vi "modbus slave全局.vi"() -> ()   [LabVIEW 2016, in "MB SLAVE.lvlib"]
uses:
  MB SLAVE.lvlib
  <vilib>/Plasmionique/MB Master/MB_Master/MB_Master.lvclass
panel:
  in  "选项卡控件":T1(tab)
  in  "与CODMn交互全局":T2 {"加标回收启动时间" format="%<%Y/%m/%d %H:%M:%S>T"; "水样启动时间" format="%<%Y/%m/%d %H:%M:%S>T"}
  in  "与氨氮交互全局":T3 {"状态告警区"."工作状态" items=["空闲"=0, "水样测试"=1, "标样核查"=2, "零点核查"=3, "跨度核查"=4, "空白测试"=5, "平行样测试"=6, "加标回收"=7, "空白校准"=8, "标样校准"=9, "初始化（清洗）"=10, "单步调试"=254, "简易流程"=255]; "状态告警区"."告警代码" items=["无告警", "缺试剂告警", "缺水样告警", "缺蒸馏水告警", "缺标液告警", "仪表漏液告警", "标定异常告警", "超量程告警", "加热异常", "低试剂预警", "超上限告警", "超下限告警", "仪表内部其他异常", "滴定异常告警", "电极异常告警", "量程切换告警", "参数设置告警", "PH电极电位异常", "电导率电极异常", "浊度光度异常", "溶解氧电极异常", "溶解氧光强异常", "温度异常告警", "PH异常告警", "溶解氧异常告警", "电导率异常告警", "浊度异常告警", "叶绿素异常告警", "藻密度异常告警", "蓝绿藻异常告警", "ORP异常告警", "氨氮异常告警", "清洁刷异常告警", "SD卡异常告警", "蓝牙异常告警", "Wifi异常告警", "流程异常告警"]; "状态告警区"."故障代码" items=["无故障", "电机故障", "温度故障", "通讯故障", "滴定故障"]}
  in  "与总磷交互全局":T4 {"状态告警区"."工作状态" items=["空闲"=0, "水样测试"=1, "标样核查"=2, "零点核查"=3, "跨度核查"=4, "空白测试"=5, "平行样测试"=6, "加标回收"=7, "空白校准"=8, "标样校准"=9, "初始化（清洗）"=10, "单步调试"=254, "简易流程"=255]; "状态告警区"."告警代码" items=["无告警", "缺试剂告警", "缺水样告警", "缺蒸馏水告警", "缺标液告警", "仪表漏液告警", "标定异常告警", "超量程告警", "加热异常", "低试剂预警", "超上限告警", "超下限告警", "仪表内部其他异常", "滴定异常告警", "电极异常告警", "量程切换告警", "参数设置告警", "PH电极电位异常", "电导率电极异常", "浊度光度异常", "溶解氧电极异常", "溶解氧光强异常", "温度异常告警", "PH异常告警", "溶解氧异常告警", "电导率异常告警", "浊度异常告警", "叶绿素异常告警", "藻密度异常告警", "蓝绿藻异常告警", "ORP异常告警", "氨氮异常告警", "清洁刷异常告警", "SD卡异常告警", "蓝牙异常告警", "Wifi异常告警", "流程异常告警"]; "状态告警区"."故障代码" items=["无故障", "电机故障", "温度故障", "通讯故障", "滴定故障"]}
  in  "与总氮交互全局":T5 {"状态告警区"."工作状态" items=["空闲"=0, "水样测试"=1, "标样核查"=2, "零点核查"=3, "跨度核查"=4, "空白测试"=5, "平行样测试"=6, "加标回收"=7, "空白校准"=8, "标样校准"=9, "初始化（清洗）"=10, "单步调试"=254, "简易流程"=255]; "状态告警区"."告警代码" items=["无告警", "缺试剂告警", "缺水样告警", "缺蒸馏水告警", "缺标液告警", "仪表漏液告警", "标定异常告警", "超量程告警", "加热异常", "低试剂预警", "超上限告警", "超下限告警", "仪表内部其他异常", "滴定异常告警", "电极异常告警", "量程切换告警", "参数设置告警", "PH电极电位异常", "电导率电极异常", "浊度光度异常", "溶解氧电极异常", "溶解氧光强异常", "温度异常告警", "PH异常告警", "溶解氧异常告警", "电导率异常告警", "浊度异常告警", "叶绿素异常告警", "藻密度异常告警", "蓝绿藻异常告警", "ORP异常告警", "氨氮异常告警", "清洁刷异常告警", "SD卡异常告警", "蓝牙异常告警", "Wifi异常告警", "流程异常告警"]; "状态告警区"."故障代码" items=["无故障", "电机故障", "温度故障", "通讯故障", "滴定故障"]}
  in  "与CODCr交互全局":T6 {"状态告警区"."工作状态" items=["空闲"=0, "水样测试"=1, "标样核查"=2, "零点核查"=3, "跨度核查"=4, "空白测试"=5, "平行样测试"=6, "加标回收"=7, "空白校准"=8, "标样校准"=9, "初始化（清洗）"=10, "单步调试"=254, "简易流程"=255]; "状态告警区"."告警代码" items=["无告警", "缺试剂告警", "缺水样告警", "缺蒸馏水告警", "缺标液告警", "仪表漏液告警", "标定异常告警", "超量程告警", "加热异常", "低试剂预警", "超上限告警", "超下限告警", "仪表内部其他异常", "滴定异常告警", "电极异常告警", "量程切换告警", "参数设置告警", "PH电极电位异常", "电导率电极异常", "浊度光度异常", "溶解氧电极异常", "溶解氧光强异常", "温度异常告警", "PH异常告警", "溶解氧异常告警", "电导率异常告警", "浊度异常告警", "叶绿素异常告警", "藻密度异常告警", "蓝绿藻异常告警", "ORP异常告警", "氨氮异常告警", "清洁刷异常告警", "SD卡异常告警", "蓝牙异常告警", "Wifi异常告警", "流程异常告警"]; "状态告警区"."故障代码" items=["无故障", "电机故障", "温度故障", "通讯故障", "滴定故障"]}
  in  "与多参数交互":T7={"pH"=TRUE, "DO"=TRUE, "Turb"=TRUE, "Cond"=TRUE, "Temp"=TRUE, "叶绿素a启用"=FALSE, "蓝绿藻"=FALSE, "藻密度"=FALSE, "orp"=FALSE}
  in  "与超标留样交互":T8
  in  "与系统交互":T9={"运行模式"=enum."维护模式", "运行间隔"=4, "流程运行中"=FALSE, "自动运行启动参数"={"氨氮"=FALSE, "总磷"=FALSE, "总氮"=FALSE, "多参数"=FALSE, "CODmn"=FALSE, "CODCr"=FALSE, "氟化物"=FALSE, "超标留样"=FALSE, "重金属"=FALSE, "挥发酚"=FALSE}, "SYSTEM Interface.总磷总氮类型"=enum."单模块", "多参数运行间隔"=4, "配水时间"=0.0, "沉淀时间"=0.0, "清洗时间"=0.0, "关键参数改变"=FALSE, "温度告警"=FALSE, "湿度告警"=FALSE, "烟感告警"=FALSE, "水浸告警"=FALSE, "开门告警"=FALSE, "SystemTask"=enum."停机", "PumpState"=enum."--", "除藻选择"=enum."不开除藻", "报警信息"=enum."无报警", "软件升级"=FALSE, "固件升级"=enum."无", "数据传输软件升级"=FALSE, "数采仪软件版本"=""} {"多参数运行间隔" min=1 max=24; "运行间隔" min=1 max=24}
  in  "Pump MB session in":refnum<class "MB_Master.lvclass">
  in  "NH3N session in":refnum<class "MB_Master.lvclass">
  in  "TP MB session in":refnum<class "MB_Master.lvclass">
  in  "TN MB session in":refnum<class "MB_Master.lvclass">
  in  "CODMn MB session in":refnum<class "MB_Master.lvclass">
  in  "CODCr MB session in":refnum<class "MB_Master.lvclass">
  in  "氟化物 MB session in":refnum<class "MB_Master.lvclass">
  in  "执行结果反馈":u16[](array[numeric])
  # "氨氮"
  # "总磷总氮"
  # "总氮"
  # "CODmn"
  # "CODCr"
  # "超标留样"
  # "多参数"
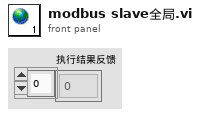
[diagram p1: front panel]
types:
  T1 = enum32{"CODMn", "氨氮", "总磷", "总氮", "CODCr", "多参数", "超标留样", "系统"}
  T2 = typedef "CODMn交互.ctl" = cluster{"COD浓度（mg/L)":dbl, "水样启动时间":timestamp, "加标回收启动时间":timestamp, "CODMn工作状态":enum16{"空闲", "水样测试", "标样核查", "零点核查", "跨度核查", "空白测试", "平行样测试", "加标回收", "空白校准", "标样校准", "初始化（清洗）"}, "多列列表框":i32, "平台试剂余量百分比":sgl, "关键参数":cluster{"测量量程":dbl, "测量精度":dbl, "测量间隔":dbl, "消解温度":dbl, "消解时长":dbl, "空白校准时间":timestamp, "曲线截距":dbl, "曲线斜率":dbl, "测量检出限":dbl, "测量信号值":dbl, "线性相关系数":dbl, "二次多项式系数":dbl, "标样校准时间":timestamp, "稀释倍数":dbl, "三项式系数":dbl, "空白标定系数":dbl, "量程系数":dbl, "F0/ORPA":dbl, "F1/ORPB":dbl, "F2/ORPK":dbl, "F3":dbl, "F4":dbl, "F5":dbl, "F6":dbl, "F7":dbl, "X0/滴定数":dbl, "量程":dbl}, "关键参数改变":bool, "校准信息":cluster{"低标液1浓度":dbl, "低标液1信号值":dbl, "低标液1启用":u16, "低标液2浓度":dbl, "低标液2信号值":dbl, "低标液2启用":u16, "低标液3浓度":dbl, "低标液3信号值":dbl, "低标液3启用":u16, "低标液4浓度":dbl, "低标液4信号值":dbl, "低标液4启用":u16, "低标液5浓度":dbl, "低标液5信号值":dbl, "低标液5启用":u16, "高标液1浓度":dbl, "高标液1信号值":dbl, "高标液1启用":u16, "高标液2浓度":dbl, "高标液2信号值":dbl, "高标液2启用":u16, "高标液3浓度":dbl, "高标液3信号值":dbl, "高标液3启用":u16, "高标液4浓度":dbl, "高标液4信号值":dbl, "高标液4启用":u16, "高标液5浓度":dbl, "高标液5信号值":dbl, "高标液5启用":u16, "低斜率":dbl, "低截距":dbl, "低二次多项式系数":dbl, "低线性相关系数":dbl, "高斜率":dbl, "高截距":dbl, "高二次多项式系数":dbl, "高线性相关系数":dbl}, "校准信息改变":bool, "固件版本号":string}
  T3 = typedef "氨氮交互.ctl" = cluster{"状态告警区":cluster{"系统时间":timestamp, "工作状态":u16, "测量模式":enum16{"待机", "连续模式", "周期模式", "定点模式", "受控模式", "手动模式"}, "告警代码":u16, "故障代码":u16, "日志代码":u16, "软件版本":u16, "F0":sgl, "F1":sgl, "F2":sgl, "F3":sgl, "T":sgl, "H":sgl, "id":u16, "flowid":u16, "量程":u16, "总磷控温温度1":sgl, "营养盐控温温度2":sgl, "ADC":sgl}, "平台试剂余量百分比":sgl, "关键参数":cluster{"测量量程":dbl, "测量精度":dbl, "测量间隔":dbl, "消解温度":dbl, "消解时长":dbl, "空白校准时间":timestamp, "曲线截距":dbl, "曲线斜率":dbl, "测量检出限":dbl, "测量信号值":dbl, "线性相关系数":dbl, "二次多项式系数":dbl, "标样校准时间":timestamp, "稀释倍数":dbl, "三项式系数":dbl, "空白标定系数":dbl, "量程系数":dbl, "F0/ORPA":dbl, "F1/ORPB":dbl, "F2/ORPK":dbl, "F3":dbl, "F4":dbl, "F5":dbl, "F6":dbl, "F7":dbl, "X0/滴定数":dbl, "量程":dbl}, "关键参数改变":bool, "校准信息":cluster{"低标液1浓度":dbl, "低标液1信号值":dbl, "低标液1启用":u16, "低标液2浓度":dbl, "低标液2信号值":dbl, "低标液2启用":u16, "低标液3浓度":dbl, "低标液3信号值":dbl, "低标液3启用":u16, "低标液4浓度":dbl, "低标液4信号值":dbl, "低标液4启用":u16, "低标液5浓度":dbl, "低标液5信号值":dbl, "低标液5启用":u16, "高标液1浓度":dbl, "高标液1信号值":dbl, "高标液1启用":u16, "高标液2浓度":dbl, "高标液2信号值":dbl, "高标液2启用":u16, "高标液3浓度":dbl, "高标液3信号值":dbl, "高标液3启用":u16, "高标液4浓度":dbl, "高标液4信号值":dbl, "高标液4启用":u16, "高标液5浓度":dbl, "高标液5信号值":dbl, "高标液5启用":u16, "低斜率":dbl, "低截距":dbl, "低二次多项式系数":dbl, "低线性相关系数":dbl, "高斜率":dbl, "高截距":dbl, "高二次多项式系数":dbl, "高线性相关系数":dbl}, "校准信息改变":bool, "固件版本号":string}
  T4 = typedef "总磷交互.ctl" = cluster{"状态告警区":cluster{"系统时间":timestamp, "工作状态":u16, "测量模式":enum16{"待机", "连续模式", "周期模式", "定点模式", "受控模式", "手动模式"}, "告警代码":u16, "故障代码":u16, "日志代码":u16, "软件版本":u16, "F0":sgl, "F1":sgl, "F2":sgl, "F3":sgl, "T":sgl, "H":sgl, "id":u16, "flowid":u16, "量程":u16, "总磷控温温度1":sgl, "营养盐控温温度2":sgl, "ADC":sgl}, "平台试剂余量百分比":sgl, "关键参数":cluster{"测量量程":dbl, "测量精度":dbl, "测量间隔":dbl, "消解温度":dbl, "消解时长":dbl, "空白校准时间":timestamp, "曲线截距":dbl, "曲线斜率":dbl, "测量检出限":dbl, "测量信号值":dbl, "线性相关系数":dbl, "二次多项式系数":dbl, "标样校准时间":timestamp, "稀释倍数":dbl, "三项式系数":dbl, "空白标定系数":dbl, "量程系数":dbl, "F0/ORPA":dbl, "F1/ORPB":dbl, "F2/ORPK":dbl, "F3":dbl, "F4":dbl, "F5":dbl, "F6":dbl, "F7":dbl, "X0/滴定数":dbl, "量程":dbl}, "关键参数改变":bool, "校准信息":cluster{"低标液1浓度":dbl, "低标液1信号值":dbl, "低标液1启用":u16, "低标液2浓度":dbl, "低标液2信号值":dbl, "低标液2启用":u16, "低标液3浓度":dbl, "低标液3信号值":dbl, "低标液3启用":u16, "低标液4浓度":dbl, "低标液4信号值":dbl, "低标液4启用":u16, "低标液5浓度":dbl, "低标液5信号值":dbl, "低标液5启用":u16, "高标液1浓度":dbl, "高标液1信号值":dbl, "高标液1启用":u16, "高标液2浓度":dbl, "高标液2信号值":dbl, "高标液2启用":u16, "高标液3浓度":dbl, "高标液3信号值":dbl, "高标液3启用":u16, "高标液4浓度":dbl, "高标液4信号值":dbl, "高标液4启用":u16, "高标液5浓度":dbl, "高标液5信号值":dbl, "高标液5启用":u16, "低斜率":dbl, "低截距":dbl, "低二次多项式系数":dbl, "低线性相关系数":dbl, "高斜率":dbl, "高截距":dbl, "高二次多项式系数":dbl, "高线性相关系数":dbl}, "校准信息改变":bool, "固件版本号":string}
  T5 = typedef "总氮交互.ctl" = cluster{"状态告警区":cluster{"系统时间":timestamp, "工作状态":u16, "测量模式":enum16{"待机", "连续模式", "周期模式", "定点模式", "受控模式", "手动模式"}, "告警代码":u16, "故障代码":u16, "日志代码":u16, "软件版本":u16, "F0":sgl, "F1":sgl, "F2":sgl, "F3":sgl, "T":sgl, "H":sgl, "id":u16, "flowid":u16, "量程":u16, "总磷控温温度1":sgl, "营养盐控温温度2":sgl, "ADC":sgl}, "平台试剂余量百分比":sgl, "关键参数":cluster{"测量量程":dbl, "测量精度":dbl, "测量间隔":dbl, "消解温度":dbl, "消解时长":dbl, "空白校准时间":timestamp, "曲线截距":dbl, "曲线斜率":dbl, "测量检出限":dbl, "测量信号值":dbl, "线性相关系数":dbl, "二次多项式系数":dbl, "标样校准时间":timestamp, "稀释倍数":dbl, "三项式系数":dbl, "空白标定系数":dbl, "量程系数":dbl, "F0/ORPA":dbl, "F1/ORPB":dbl, "F2/ORPK":dbl, "F3":dbl, "F4":dbl, "F5":dbl, "F6":dbl, "F7":dbl, "X0/滴定数":dbl, "量程":dbl}, "关键参数改变":bool, "校准信息":cluster{"低标液1浓度":dbl, "低标液1信号值":dbl, "低标液1启用":u16, "低标液2浓度":dbl, "低标液2信号值":dbl, "低标液2启用":u16, "低标液3浓度":dbl, "低标液3信号值":dbl, "低标液3启用":u16, "低标液4浓度":dbl, "低标液4信号值":dbl, "低标液4启用":u16, "低标液5浓度":dbl, "低标液5信号值":dbl, "低标液5启用":u16, "高标液1浓度":dbl, "高标液1信号值":dbl, "高标液1启用":u16, "高标液2浓度":dbl, "高标液2信号值":dbl, "高标液2启用":u16, "高标液3浓度":dbl, "高标液3信号值":dbl, "高标液3启用":u16, "高标液4浓度":dbl, "高标液4信号值":dbl, "高标液4启用":u16, "高标液5浓度":dbl, "高标液5信号值":dbl, "高标液5启用":u16, "低斜率":dbl, "低截距":dbl, "低二次多项式系数":dbl, "低线性相关系数":dbl, "高斜率":dbl, "高截距":dbl, "高二次多项式系数":dbl, "高线性相关系数":dbl}, "校准信息改变":bool, "固件版本号":string}
  T6 = typedef "CODCr交互.ctl" = cluster{"状态告警区":cluster{"系统时间":timestamp, "工作状态":u16, "测量模式":enum16{"待机", "连续模式", "周期模式", "定点模式", "受控模式", "手动模式"}, "告警代码":u16, "故障代码":u16, "日志代码":u16, "软件版本":u16, "F0":sgl, "F1":sgl, "F2":sgl, "F3":sgl, "T":sgl, "H":sgl, "id":u16, "flowid":u16, "量程":u16, "总磷控温温度1":sgl, "营养盐控温温度2":sgl, "ADC":sgl}, "平台试剂余量百分比":sgl, "关键参数":cluster{"测量量程":dbl, "测量精度":dbl, "测量间隔":dbl, "消解温度":dbl, "消解时长":dbl, "空白校准时间":timestamp, "曲线截距":dbl, "曲线斜率":dbl, "测量检出限":dbl, "测量信号值":dbl, "线性相关系数":dbl, "二次多项式系数":dbl, "标样校准时间":timestamp, "稀释倍数":dbl, "三项式系数":dbl, "空白标定系数":dbl, "量程系数":dbl, "F0/ORPA":dbl, "F1/ORPB":dbl, "F2/ORPK":dbl, "F3":dbl, "F4":dbl, "F5":dbl, "F6":dbl, "F7":dbl, "X0/滴定数":dbl, "量程":dbl}, "关键参数改变":bool, "校准信息":cluster{"低标液1浓度":dbl, "低标液1信号值":dbl, "低标液1启用":u16, "低标液2浓度":dbl, "低标液2信号值":dbl, "低标液2启用":u16, "低标液3浓度":dbl, "低标液3信号值":dbl, "低标液3启用":u16, "低标液4浓度":dbl, "低标液4信号值":dbl, "低标液4启用":u16, "低标液5浓度":dbl, "低标液5信号值":dbl, "低标液5启用":u16, "高标液1浓度":dbl, "高标液1信号值":dbl, "高标液1启用":u16, "高标液2浓度":dbl, "高标液2信号值":dbl, "高标液2启用":u16, "高标液3浓度":dbl, "高标液3信号值":dbl, "高标液3启用":u16, "高标液4浓度":dbl, "高标液4信号值":dbl, "高标液4启用":u16, "高标液5浓度":dbl, "高标液5信号值":dbl, "高标液5启用":u16, "低斜率":dbl, "低截距":dbl, "低二次多项式系数":dbl, "低线性相关系数":dbl, "高斜率":dbl, "高截距":dbl, "高二次多项式系数":dbl, "高线性相关系数":dbl}, "校准信息改变":bool, "固件版本号":string}
  T7 = typedef "多参数交互.ctl" = cluster{"pH":bool, "DO":bool, "Turb":bool, "Cond":bool, "Temp":bool, "叶绿素a启用":bool, "蓝绿藻":bool, "藻密度":bool, "orp":bool}
  T8 = typedef "超标留样交互.ctl" = cluster{"当前瓶号":u16}
  T9 = typedef "系统交互.ctl" = cluster{"运行模式":enum16{"维护模式", "常规模式", "应急模式", "质控模式", "性能测试"}, "运行间隔":i16, "流程运行中":bool, "自动运行启动参数":T10, "SYSTEM Interface.总磷总氮类型":enum16{"单模块", "总磷总氮二合一模块", "氨氮总磷二合一模块"}, "多参数运行间隔":i16, "配水时间":dbl, "沉淀时间":dbl, "清洗时间":dbl, "关键参数改变":bool, "温度告警":bool, "湿度告警":bool, "烟感告警":bool, "水浸告警":bool, "开门告警":bool, "SystemTask":enum16{"停机", "待机", "调试", "水样采集", "沉沙", "进样", "仪表测试分析", "反吹", "清洗", "除藻"}, "PumpState":enum16{"--", "只用泵1", "只用泵2", "双泵交替"}, "除藻选择":enum16{"不开除藻", "开除藻"}, "报警信息":enum16{"无报警", "断电报警", "采样管理欠压（源水泵故障）", "进样管路欠压（进样泵/增加泵故障）"}, "软件升级":bool, "固件升级":enum16{"无", "CODMn", "氨氮", "总磷", "总氮", "CODCr"}, "数据传输软件升级":bool, "数采仪软件版本":string}
  T10 = typedef "启动参数.ctl" = cluster{"氨氮":bool, "总磷":bool, "总氮":bool, "多参数":bool, "CODmn":bool, "CODCr":bool, "氟化物":bool, "超标留样":bool, "重金属":bool, "挥发酚":bool}
diagram:
